vi "Configure Active Phase.vi"(0 "VISA resource name":refnum<visa-resource-name>, 5 "Output Phase(s) (3-Phase)":u16(ring)=3 items=["1-Phase"=1, "3-Phase"=3], 7 "Enable Coupling (Enabled)":bool=TRUE, 9 "Active Phase (1:Phase 1)":i32(ring)=1 items=["Phase 1"=1, "Phase 2"=2, "Phase 3"=3], 11 "error in (no error)":errorcluster) -> (4 "VISA resource name out":refnum<visa-resource-name>, 15 "error out":errorcluster)   [LabVIEW 2011, in "California Instruments iX Series.lvlib"]
doc: "Configures the three phase output capability of the AC Power Source. \n\n<b>Note:</b>\nThis VI does not support single phase output models. Single phase units always operate on Phase A only."
uses:
  <instrlib>/California Instruments iX Series/California Instruments iX Series.lvlib
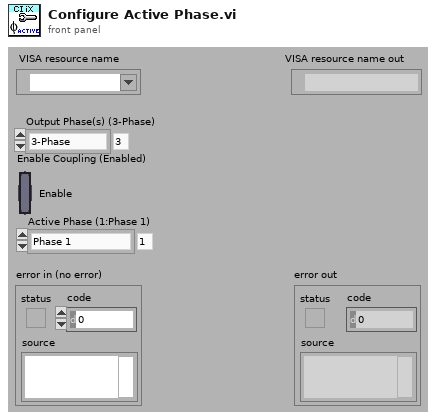
[diagram p1: front panel]
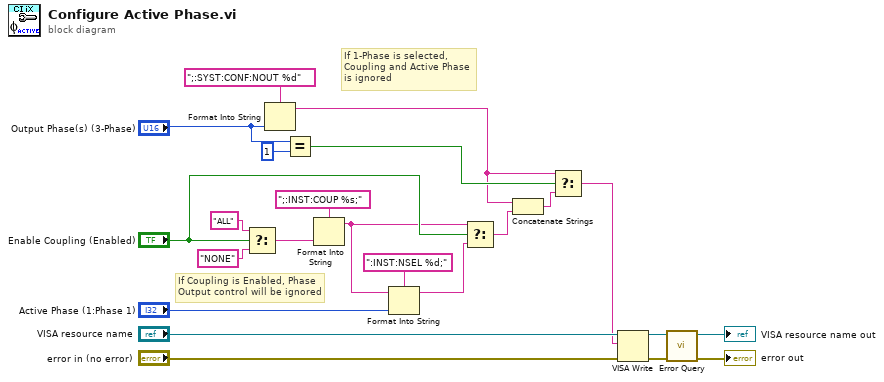
[diagram p0: block diagram]
diagram:
  # "If 1-Phase is selected, Coupling and Active Phase is ignored"
  # "If Coupling is Enabled, Phase Output control will be ignored"
  n1 = Select(t="ALL", s="Enable Coupling (Enabled)", f="NONE") -> (s? t:f=w14:string)
  n2 = Format Into String(format string=";:SYST:CONF:NOUT %d", "Output Phase(s) (3-Phase)") -> (resulting string=w4:string)  [unwired: 2 in, 1 out]
  n3 = Equal?(x="Output Phase(s) (3-Phase)", y=u16 1) -> (x = y?=w5:bool)
  n4 = Format Into String(format string=";:INST:COUP %s;", w14) -> (resulting string=w10:string)  [unwired: 2 in, 1 out]
  n5 = Format Into String(format string=":INST:NSEL %d;", initial string=w10, "Active Phase (1:Phase 1)") -> (resulting string=w9:string)  [unwired: 1 in, 1 out]
  n6 = Select(t=w10, s="Enable Coupling (Enabled)", f=w9) -> (s? t:f=w3:string)
  n7 = Concatenate Strings(w4, w3) -> (w2:string)
  n8 = Select(t=w4, s=w5, f=w2) -> (s? t:f=w1:string)
  n9 = VISA Write(VISA resource name="VISA resource name", write buffer=w1, error in (no error)="error in (no error)") -> (VISA resource name out=w21:refnum<visa-resource-name>, error out=w20:errorcluster)  [unwired: 1 out]
  n10 = call <instrlib>:"Error Query.vi"("error in (no error)"=w20, "VISA resource name"=w21) -> ("error out"=→"error out":errorcluster, "VISA resource name out"=→"VISA resource name out":refnum<visa-resource-name>)  [unwired: 6 in, 2 out]
